vi "Inspect.vi"(10 "Msg Strategy in":refnum<class "Msg Strategy.lvclass">, 11 "jettl in":refnum<class "jettl.lvclass">) -> (2 "Msg Strategy out":refnum<class "Msg Strategy.lvclass">, 3 "jettl out":refnum<class "jettl.lvclass">)   [LabVIEW 2021, in "jettl.lvlib" / "jettl.lvclass"]
uses:
  jettl.lvclass
  Msg Strategy/Msg Strategy.lvclass
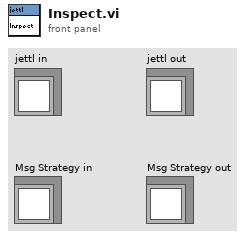
[diagram p1: front panel]
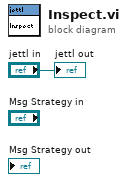
[diagram p0: block diagram]
diagram:
  "jettl out" <- "jettl in"
